vi "Node_ID_AlarmWarning.vi"(8 "error in":errorcluster) -> (0 "error out":errorcluster, 1 "node RU 3":string[](array[string]), 2 "node RU 2":T1[](array[typedef]), 3 "node RU":T1[](array[typedef]))   [LabVIEW 2019]
uses:
  <vilib>/OPCUA/controls/NodeId.ctl
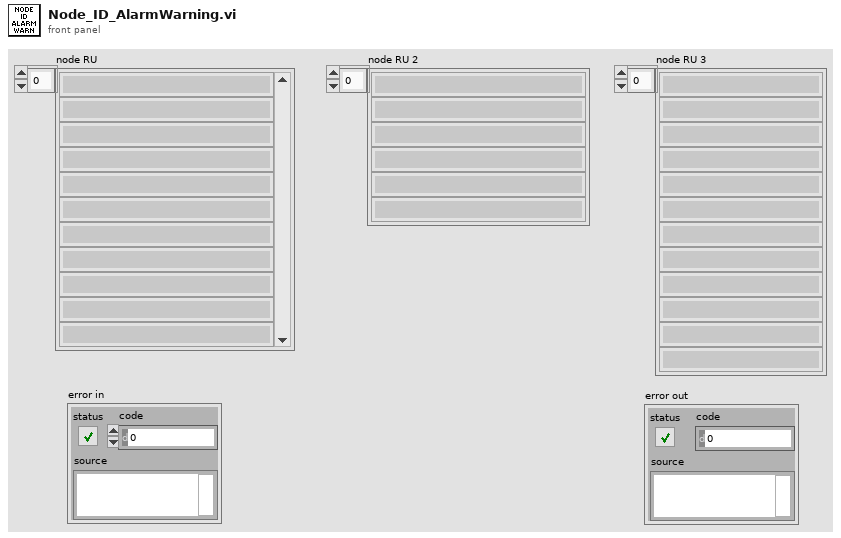
[diagram p1: front panel]
types:
  T1 = typedef "NodeId.ctl" = string
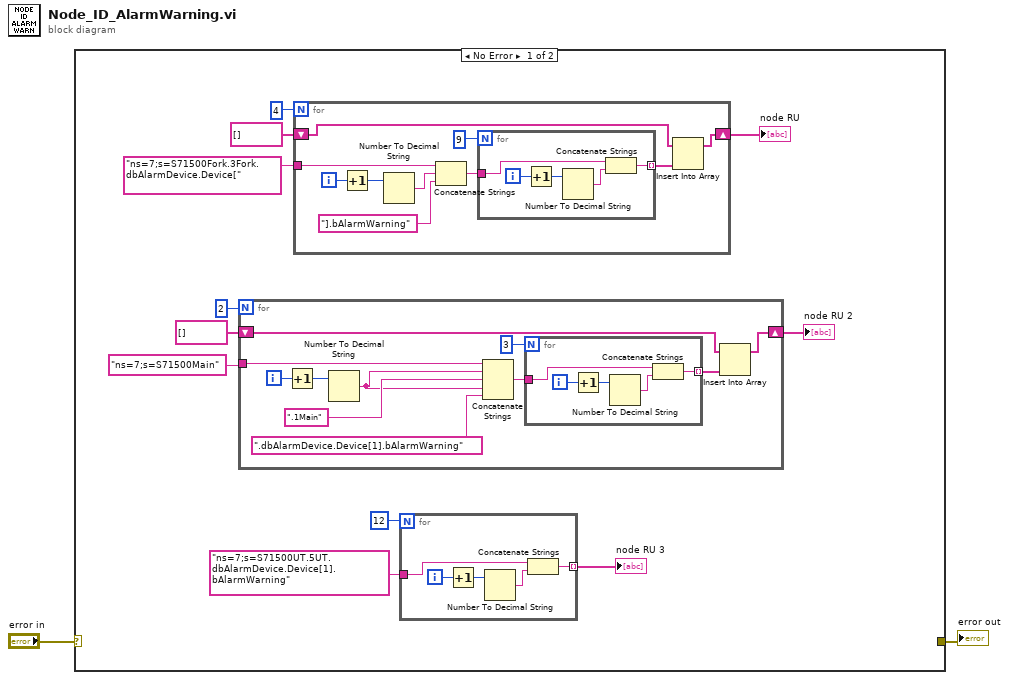
[diagram p0: block diagram]
diagram:
  n1 = case shown="No Error" "error in" {
    selector: "error in" -> [_ w50]
    tunnel: [_ w50] -> w1
    frame No Error {
      n2 = for {
        N: 2 -> [_]
        tunnel: T1 "ns=7;s=S71500Main" ("node RU") -> [w28]
        shift-right: [w25] -> w6
        shift-left: T1[] [] ("node RU") -> [w23]
        i -> [w27]
        n3 = Increment(x=w27) -> (x+1=w29:i32)
        n4 = Number To Decimal String(number=w29) -> (decimal integer string=w21:string)  [unwired: 1 in]
        n5 = Concatenate Strings(w28, w21, ".1Main" ("string"), w21, ".dbAlarmDevice.Device[1].bAlarmWarning" ("string")) -> (w26:string)
        n6 = for {
          N: 3 -> [_]
          tunnel: w26 -> [w34]
          tunnel: [w30] -> w24 mode=indexing
          i -> [w33]
          n7 = Increment(x=w33) -> (x+1=w32:i32)
          n8 = Number To Decimal String(number=w32) -> (decimal integer string=w31:string)  [unwired: 1 in]
          n9 = Concatenate Strings(w34, w31) -> (w30:string)
        }
        n10 = Insert Into Array(array=w23, new element=w24) -> (w25:T1[])  [unwired: 1 in]
      }
      "node RU 2" <- w6
      n11 = for {
        N: 4 -> [_]
        tunnel: T1 "ns=7;s=S71500Fork.3Fork.dbAlarmDevice.Device[" ("node RU") -> [w42]
        shift-right: [w37] -> w10
        shift-left: T1[] [] ("node RU") -> [w35]
        i -> [w41]
        n12 = Increment(x=w41) -> (x+1=w44:i32)
        n13 = Number To Decimal String(number=w44) -> (decimal integer string=w43:string)  [unwired: 1 in]
        n14 = Concatenate Strings(w42, w43, "].bAlarmWarning" ("string")) -> (w38:string)
        n15 = for {
          N: 9 -> [_]
          tunnel: w38 -> [w49]
          tunnel: [w45] -> w36 mode=indexing
          i -> [w48]
          n16 = Increment(x=w48) -> (x+1=w47:i32)
          n17 = Number To Decimal String(number=w47) -> (decimal integer string=w46:string)  [unwired: 1 in]
          n18 = Concatenate Strings(w49, w46) -> (w45:string)
        }
        n19 = Insert Into Array(array=w35, new element=w36) -> (w37:T1[])  [unwired: 1 in]
      }
      "node RU" <- w10
      n20 = for {
        N: 12 -> [_]
        tunnel: T1 "ns=7;s=S71500UT.5UT.dbAlarmDevice.Device[1].bAlarmWarning" ("node RU") -> [w18]
        tunnel: [w14] -> w3 mode=indexing
        i -> [w17]
        n21 = Increment(x=w17) -> (x+1=w16:i32)
        n22 = Number To Decimal String(number=w16) -> (decimal integer string=w15:string)  [unwired: 1 in]
        n23 = Concatenate Strings(w18, w15) -> (w14:string)
      }
      "node RU 3" <- w3
    }
    frame Error {
    }
  }
  "error out" <- w1
